vi "DriveModuleNetwork.vi"(8 "error in (no error)":errorcluster, 11 "Module":i32) -> (0 "error out":errorcluster)   [LabVIEW 2023]
doc: "Network for Drive\n\nInputs:\n -- Error in -- Error cluster -- propagated error input\n\nOutputs:\n -- Error out -- Error cluster -- progated error output"
uses:
  DriveGlobal.vi
  <vilib>/Rock Robotics/Network Tables/NT Write Number.vi
  <vilib>/Rock Robotics/WPI/ThirdParty/JAS_Junk/TrajLib/Trajectory_Library.lvlib
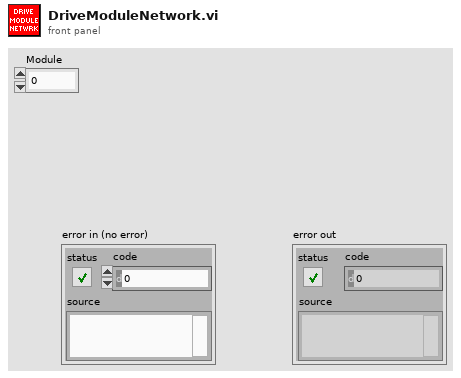
[diagram p1: front panel]
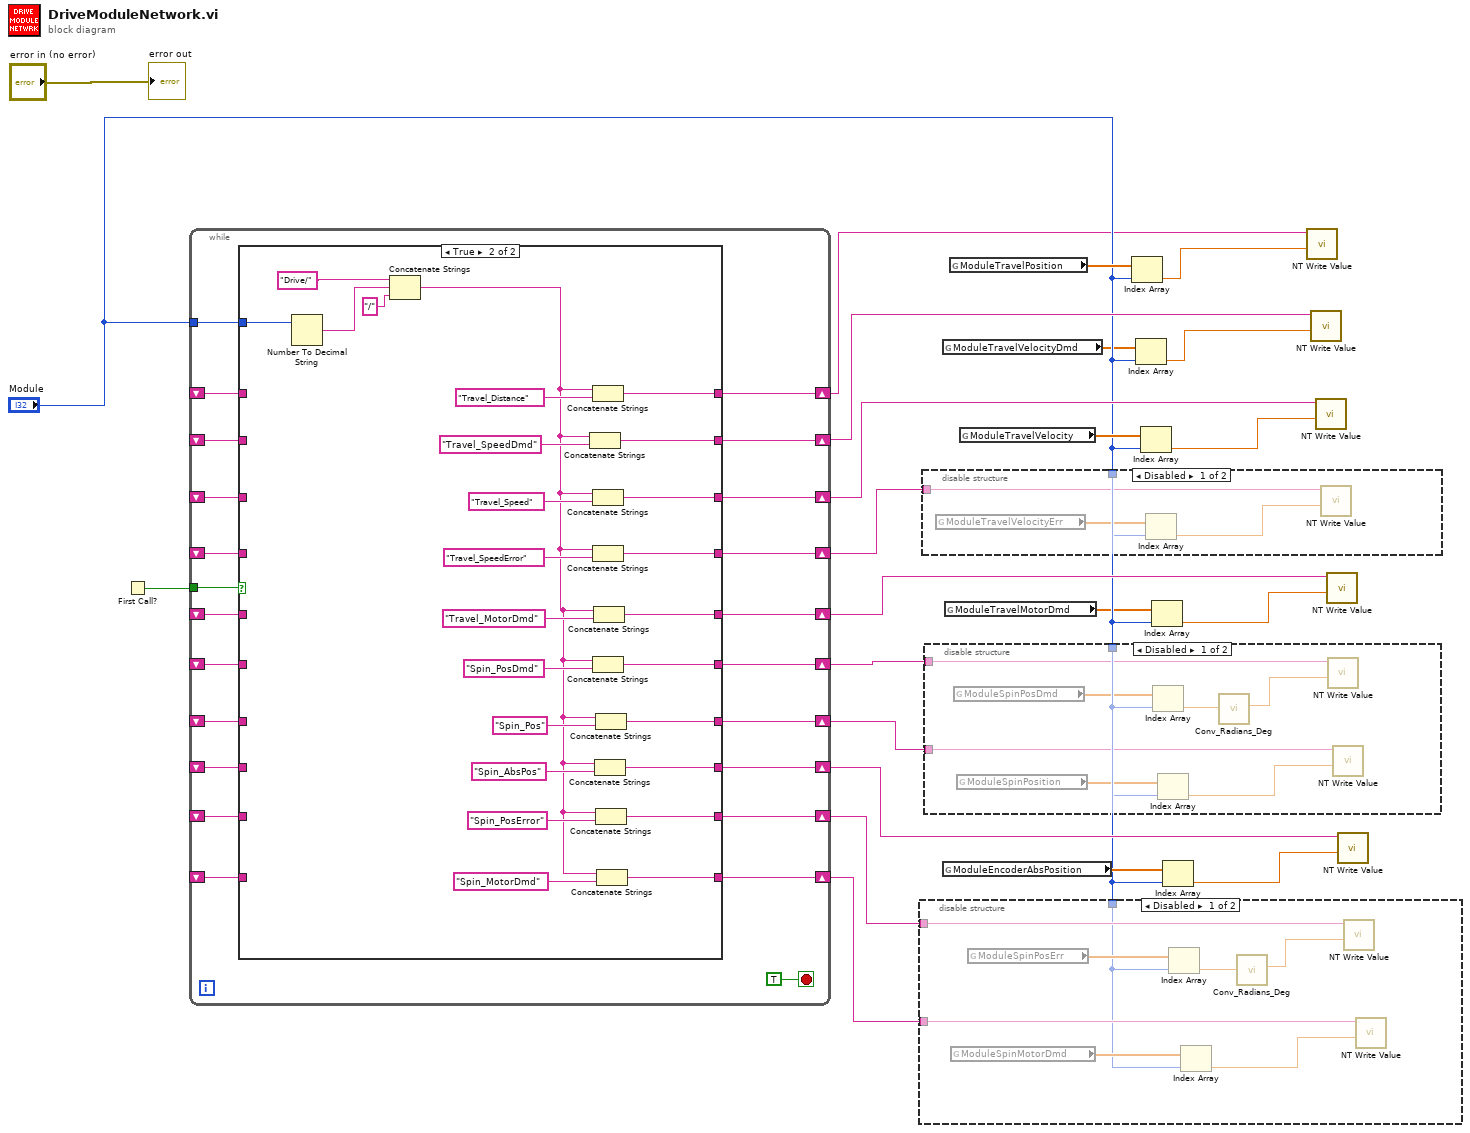
[diagram p0: block diagram]
diagram:
  n1 = First Call?() -> (First Call?: T/F=w22:bool)
  n2 = while {
    tunnel: w22 -> [w45]
    tunnel: "Module" -> [w44]
    shift-right: [w43] -> w21
    shift-left: _ -> [w34]
    shift-right: [w42] -> w16
    shift-left: _ -> [w33]
    shift-right: [w41] -> w15
    shift-left: _ -> [w31]
    shift-right: [w40] -> w14
    shift-left: _ -> [w32]
    shift-right: [w39] -> w13
    shift-left: _ -> [w30]
    shift-right: [w38] -> w12
    shift-left: _ -> [w29]
    shift-right: [w37] -> w11
    shift-left: _ -> [w28]
    shift-right: [w36] -> w10
    shift-left: _ -> [w27]
    shift-right: [w35] -> w9
    shift-left: _ -> [w26]
    shift-right: [w25] -> w5
    shift-left: _ -> [w24]
    stop <- TRUE stop-if-true
    n3 = case shown="True" w45 {
      tunnel: w44 -> [_ w80]
      tunnel: [w56 w68] -> w43
      tunnel: [w55 w67] -> w42
      tunnel: [w53 w66] -> w41
      tunnel: [w54 w65] -> w40
      tunnel: [w52 w64] -> w39
      tunnel: [w51 w63] -> w38
      tunnel: [w50 w62] -> w37
      tunnel: [w49 w61] -> w36
      tunnel: [w48 w60] -> w35
      tunnel: w34 -> [w56 _]
      tunnel: w33 -> [w55 _]
      tunnel: w32 -> [w54 _]
      tunnel: w31 -> [w53 _]
      tunnel: w30 -> [w52 _]
      tunnel: w29 -> [w51 _]
      tunnel: w28 -> [w50 _]
      tunnel: w27 -> [w49 _]
      tunnel: w26 -> [w48 _]
      tunnel: [w47 w57] -> w25
      tunnel: w24 -> [w47 _]
      frame False {
      }
      frame True {
        n4 = Number To Decimal String(number=w80) -> (decimal integer string=w79:string)  [unwired: 1 in]
        n5 = Concatenate Strings("Drive/", w79, "/" ("string")) -> (w58:string)
        n6 = Concatenate Strings(w58, "Travel_SpeedDmd" ("string")) -> (w68:string)
        n7 = Concatenate Strings(w58, "Travel_Distance" ("string")) -> (w57:string)
        n8 = Concatenate Strings(w58, "Travel_Speed" ("string")) -> (w67:string)
        n9 = Concatenate Strings(w58, "Travel_SpeedError" ("string")) -> (w66:string)
        n10 = Concatenate Strings(w58, "Spin_PosDmd" ("string")) -> (w64:string)
        n11 = Concatenate Strings(w58, "Travel_MotorDmd" ("string")) -> (w65:string)
        n12 = Concatenate Strings(w58, "Spin_AbsPos" ("string")) -> (w62:string)
        n13 = Concatenate Strings(w58, "Spin_Pos" ("string")) -> (w63:string)
        n14 = Concatenate Strings(w58, "Spin_PosError" ("string")) -> (w61:string)
        n15 = Concatenate Strings(w58, "Spin_MotorDmd" ("string")) -> (w60:string)
      }
    }
  }
  n16 = disable-structure shown="Disabled" {
    disable-tunnel: w10 -> [w86 _]
    disable-tunnel: w9 -> [w85 _]
    disable-tunnel: "Module" -> [w84 _]
    frame Disabled {
      n17 = global read "DriveGlobal.vi" "ModuleSpinMotorDmd"() -> (w88:dbl[])
      n18 = global read "DriveGlobal.vi" "ModuleSpinPosErr"() -> (w89:dbl[])
      n19 = Index Array(array=w89, index=w84) -> (element=w83:dbl)
      n20 = Index Array(array=w88, index=w84) -> (element=w87:dbl)
      n21 = call <vilib>:"Conv_Radians_Deg.vi"("Radians"=w83) -> ("Degrees"=w82:dbl)  [unwired: 10 in]
      n22 = call-poly <vilib>:"NT Write Value.vi"("value"=w82, "name"=w86) -> ()  [unwired: 9 in, 1 out]
      n23 = call-poly <vilib>:"NT Write Value.vi"("value"=w87, "name"=w85) -> ()  [unwired: 9 in, 1 out]
    }
    frame Enabled {
    }
  }
  n24 = disable-structure shown="Disabled" {
    disable-tunnel: w15 -> [w93 _]
    disable-tunnel: "Module" -> [w92 _]
    frame Disabled {
      n25 = global read "DriveGlobal.vi" "ModuleTravelVelocityErr"() -> (w91:dbl[])
      n26 = Index Array(array=w91, index=w92) -> (element=w90:dbl)
      n27 = call-poly <vilib>:"NT Write Value.vi"("value"=w90, "name"=w93) -> ()  [unwired: 9 in, 1 out]
    }
    frame Enabled {
    }
  }
  n28 = disable-structure shown="Disabled" {
    disable-tunnel: w13 -> [w101 _]
    disable-tunnel: w12 -> [w100 _]
    disable-tunnel: "Module" -> [w99 _]
    frame Disabled {
      n29 = global read "DriveGlobal.vi" "ModuleSpinPosDmd"() -> (w98:dbl[])
      n30 = global read "DriveGlobal.vi" "ModuleSpinPosition"() -> (w97:dbl[])
      n31 = Index Array(array=w98, index=w99) -> (element=w95:dbl)
      n32 = Index Array(array=w97, index=w99) -> (element=w96:dbl)
      n33 = call <vilib>:"Conv_Radians_Deg.vi"("Radians"=w95) -> ("Degrees"=w94:dbl)  [unwired: 10 in]
      n34 = call-poly <vilib>:"NT Write Value.vi"("value"=w94, "name"=w101) -> ()  [unwired: 9 in, 1 out]
      n35 = call-poly <vilib>:"NT Write Value.vi"("value"=w96, "name"=w100) -> ()  [unwired: 9 in, 1 out]
    }
    frame Enabled {
    }
  }
  n36 = global read "DriveGlobal.vi" "ModuleTravelVelocityDmd"() -> (w4:dbl[])
  n37 = global read "DriveGlobal.vi" "ModuleEncoderAbsPosition"() -> (w18:dbl[])
  n38 = global read "DriveGlobal.vi" "ModuleTravelMotorDmd"() -> (w2:dbl[])
  n39 = global read "DriveGlobal.vi" "ModuleTravelPosition"() -> (w8:dbl[])
  n40 = global read "DriveGlobal.vi" "ModuleTravelVelocity"() -> (w20:dbl[])
  n41 = Index Array(array=w8, index="Module") -> (element=w7:dbl)
  n42 = Index Array(array=w4, index="Module") -> (element=w3:dbl)
  n43 = Index Array(array=w20, index="Module") -> (element=w19:dbl)
  n44 = Index Array(array=w2, index="Module") -> (element=w1:dbl)
  n45 = Index Array(array=w18, index="Module") -> (element=w17:dbl)
  n46 = call-poly <vilib>:"NT Write Value.vi"("value"=w7, "name"=w5) -> ()  [unwired: 9 in, 1 out]
  n47 = call-poly <vilib>:"NT Write Value.vi"("value"=w3, "name"=w21) -> ()  [unwired: 9 in, 1 out]
  n48 = call-poly <vilib>:"NT Write Value.vi"("value"=w19, "name"=w16) -> ()  [unwired: 9 in, 1 out]
  n49 = call-poly <vilib>:"NT Write Value.vi"("value"=w1, "name"=w14) -> ()  [unwired: 9 in, 1 out]
  n50 = call-poly <vilib>:"NT Write Value.vi"("value"=w17, "name"=w11) -> ()  [unwired: 9 in, 1 out]
  "error out" <- "error in (no error)"
